vi "tlc_error_main.vi"(7 "Command (Check Error)":T1=enum."Check Error", 8 "error in (no error)":errorcluster, 10 "Error User Event Refnum":T3, 11 "Consumer Queue Refnum":T2) -> (0 "error out":errorcluster)   [LabVIEW 2009]
uses:
  controls/tlc_ErrorUserEvent_refnum.ctl
  controls/tlc_ConsumerQueue_refnum.ctl
  controls/tlc_ConsumerDataType_enum.ctl
  controls/tlc_ConsumerCommand_enum.ctl
  tlc_error_Command_enum.ctl
panel:
  # "Inputs"
  # "Outputs"
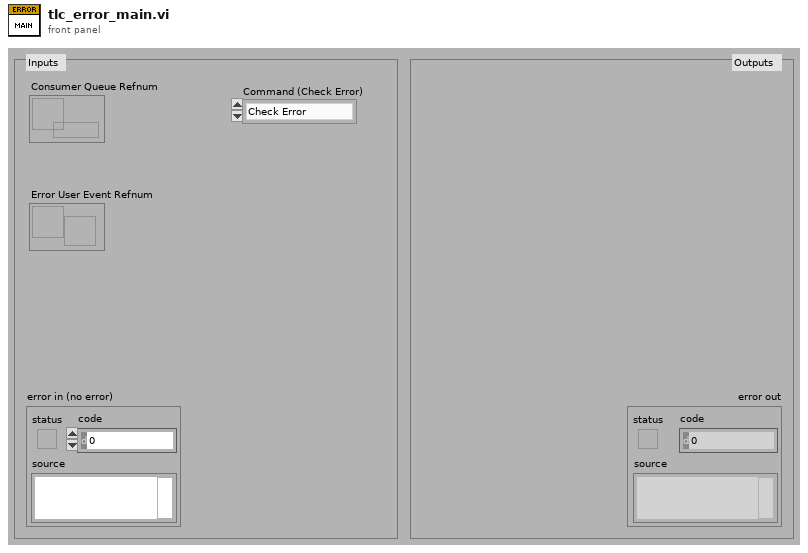
[diagram p1: front panel]
types:
  T1 = typedef "tlc_error_Command_enum.ctl" = enum16{"Initialise", "Check Error", "Report Errors"}
  T2 = typedef "tlc_ConsumerQueue_refnum.ctl" = refnum<queue>
  T3 = typedef "tlc_ErrorUserEvent_refnum.ctl" = refnum<user-event>
  T4 = typedef "tlc_ConsumerDataType_enum.ctl" = cluster{"Command":T5, "Data":variant}
  T5 = typedef "tlc_ConsumerCommand_enum.ctl" = enum16{"Initialise", "Check Controller", "Exit"}
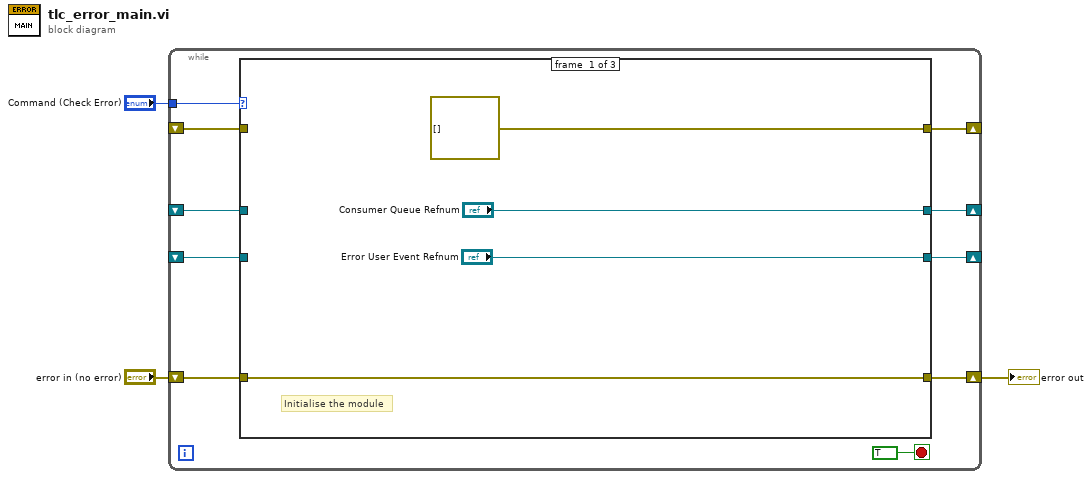
[diagram p0: block diagram]
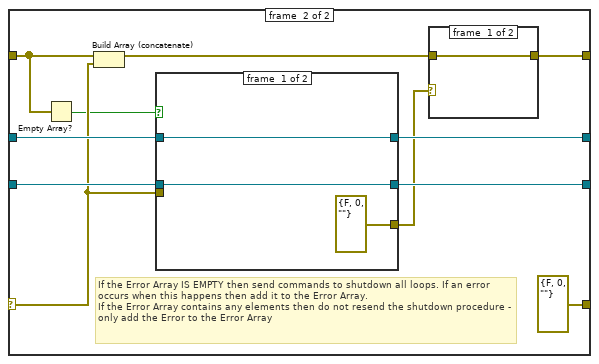
[diagram p3: hidden frame]
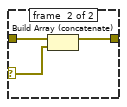
[diagram p4: hidden frame]
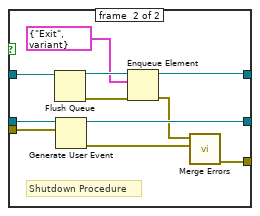
[diagram p5: hidden frame]
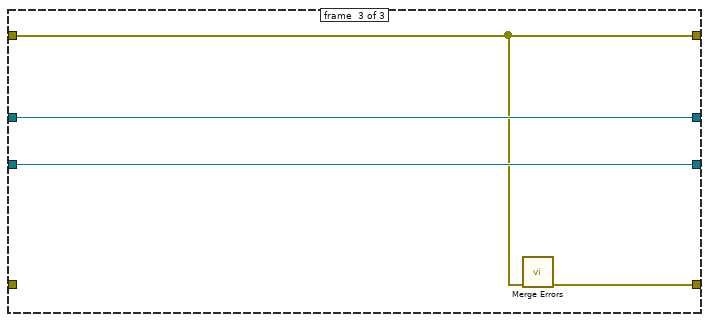
[diagram p6: hidden frame]
diagram:
  n1 = while {
    shift-right: [w13] -> w2
    shift-left: "error in (no error)" -> [w12]
    tunnel: "Command (Check Error)" -> [w11]
    shift-right: [w9] -> _
    shift-left: _ -> [w7]
    shift-right: [w8] -> _
    shift-left: _ -> [w6]
    shift-right: [w5] -> _
    shift-left: _ -> [w4]
    stop <- TRUE stop-if-true
    n2 = case shown="\"Check Error\"" w11 {
      tunnel: [w17 w18 w59] -> w13
      tunnel: w12 -> [w17 w25 _]
      tunnel: ["Consumer Queue Refnum" w20 w62] -> w9
      tunnel: ["Error User Event Refnum" w19 w61] -> w8
      tunnel: w7 -> [_ w24 w62]
      tunnel: w6 -> [_ w23 w61]
      tunnel: [errorcluster[] [] w21 w60] -> w5
      tunnel: w4 -> [_ w22 w60]
      frame #0 {
        # "Initialise the module"
      }
      frame #1 {
        n3 = case shown="Error" w25 {
          selector: w25 -> [w26 w33]
          tunnel: w24 -> [w28 w40]
          tunnel: w23 -> [w27 w39]
          tunnel: w22 -> [w29 w31]
          tunnel: [w29 w35] -> w21
          tunnel: [w28 w37] -> w20
          tunnel: [w27 w38] -> w19
          tunnel: [w26 errorcluster {"status"=FALSE, "code"=0, "source"=""} ("error out")] -> w18
          frame #0 {
            # "No Error - do nothing"
          }
          frame #1 {
            # "If the Error Array IS EMPTY then send commands to shutdown all loops. If an error occurs when this happens then add it to the Error Array.\nIf the Error Array contains any elements then do not resend the shutdown procedure - only add the Error to the Error Array"
            n4 = Empty Array?(array=w31) -> (empty?=w30:bool)
            n5 = Build Array (concatenate)(w31, w33) -> (w34:errorcluster[])
            n6 = case shown="True" w30 {
              tunnel: w40 -> [w46 w54]
              tunnel: w39 -> [w47 w56]
              tunnel: w33 -> [_ w57]
              tunnel: [w47 w55] -> w38
              tunnel: [w46 w53] -> w37
              tunnel: [errorcluster {"status"=FALSE, "code"=0, "source"=""} ("error IO") w48] -> w36
              frame #0 {
              }
              frame #1 {
                # "Shutdown Procedure"
                n7 = Flush Queue(queue=w54) -> (queue out=w52:T2, error out=w58:errorcluster)  [unwired: 1 in, 1 out]
                n8 = Generate User Event(user event=w56, event data cluster=w57) -> (user event out=w55:T3, error out=w49:errorcluster)  [unwired: 1 in]
                n9 = Enqueue Element(queue=w52, element=T4 {"Command"=enum."Exit", "Data"=variant}, error in (no error)=w58) -> (queue out=w53:T2, error out=w50:errorcluster)  [unwired: 1 in, 1 out]
                n10 = call <vilib>:"Merge Errors.vi"("error in 2 (no error)"=w49, "error in 1 (no error)"=w50) -> ("error out"=w48:errorcluster)  [unwired: 5 in]
              }
            }
            n11 = case shown="Error" w36 {
              selector: w36 -> [_ w42]
              tunnel: [w41 w43] -> w35
              tunnel: w34 -> [w41 w44]
              frame #0 {
              }
              frame #1 {
                n12 = Build Array (concatenate)(w44, w42) -> (w43:errorcluster[])
              }
            }
          }
        }
      }
      frame #2 {
        n13 = call <vilib>:"Merge Errors.vi"("error array in"=w60) -> ("error out"=w59:errorcluster)  [unwired: 6 in]
      }
    }
  }
  "error out" <- w2
